vi "Discovery Management.vi"(11 "CIFPluginManager in":refnum<class "CIFPluginManager.lvclass">) -> (0 "error out":errorcluster)   [LabVIEW 2021, in "CIFPluginManager.lvclass"]
uses:
  CIFPluginManager.lvclass
  typedef/Discover Command.ctl
  CIFUtilities/CIFLogs/CIFLogs.lvlib
  gRPC/CIF_Manager_Client_Wrapper/CIFManagerClientWrapper.lvlib
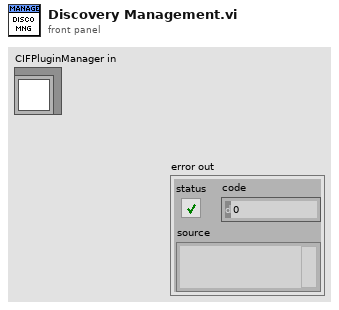
[diagram p1: front panel]
types:
  T1 = typedef "CIFPluginManager.lvclass/Discover Command.ctl" = cluster{"Loader Name":string, "Update Metadata":bool}
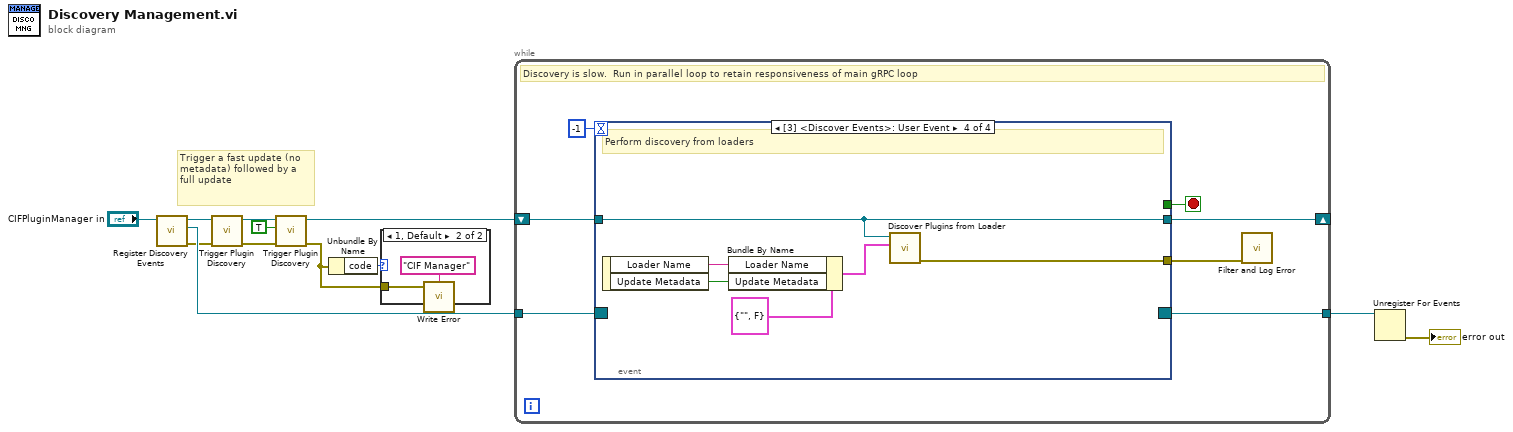
[diagram p0: block diagram]
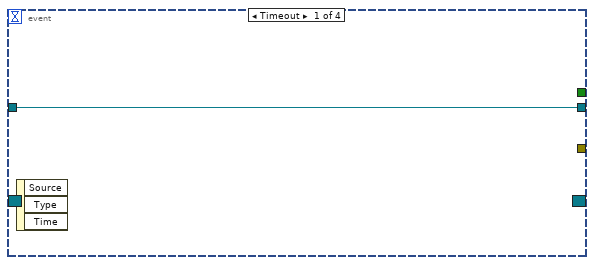
[diagram p3: hidden frame]
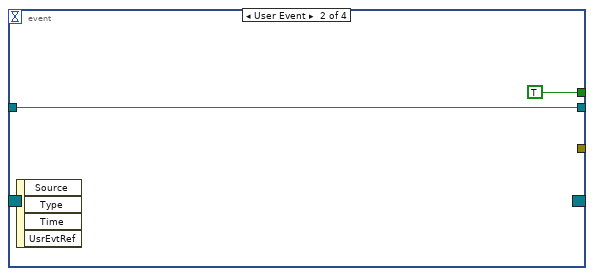
[diagram p4: hidden frame]
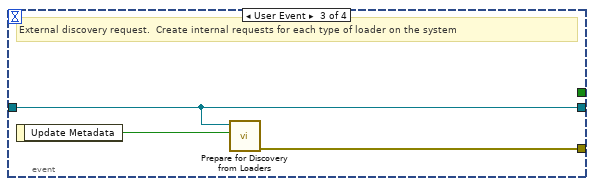
[diagram p5: hidden frame]
diagram:
  # "Trigger a fast update (no metadata) followed by a full update"
  n1 = call "Register Discovery Events.vi"("CIFPluginManager in"="CIFPluginManager in") -> ("error out"=w7:errorcluster, "Event Registration Refnum"=w9:refnum<event-registration>, "CIFPluginManager out"=w6:refnum<class "CIFPluginManager.lvclass">)  [unwired: 8 in]
  n2 = call "Trigger Plugin Discovery.vi"("error in (no error)"=w7, "CIFPluginManager in"=w6) -> ("error out"=w4:errorcluster, "CIFPluginManager out"=w5:refnum<class "CIFPluginManager.lvclass">)  [unwired: 8 in]
  n3 = call "Trigger Plugin Discovery.vi"("error in (no error)"=w4, "Update Metadata"=TRUE, "CIFPluginManager in"=w5) -> ("error out"=w2:errorcluster, "CIFPluginManager out"=w3:refnum<class "CIFPluginManager.lvclass">)  [unwired: 7 in]
  n4 = Unbundle By Name(w2) -> ("code"=w10:i32)
  n5 = case shown="1, Default" w10 {
    tunnel: w2 -> [_ w14]
    frame 0 {
      # "-1001 is cancelled by client.  Not an error."
    }
    frame 1, Default {
      n6 = call "Write Error.vi"("error in (no error)"=w14, "Plugin Name"="CIF Manager") -> ()  [unwired: 2 in, 1 out]
    }
  }
  n7 = while {
    tunnel: w9 -> [w15]
    shift-right: [w19] -> _
    shift-left: w3 -> [w21]
    tunnel: [w17] -> w11
    stop <- w18 stop-if-true
    # "Discovery is slow.  Run in parallel loop to retain responsiveness of main gRPC loop"
    n8 = event shown="[3] <Discover Events>: User Event" {
      selector: w15 -> [_ _ _ _]
      dyn-events: [_ _ _ _] -> w17
      timeout: -1 -> [_ _ _ _]
      tunnel: w21 -> [w22 w23 w26 w32]
      tunnel: [w22 w23 w26 w32] -> w19
      tunnel: [_ TRUE _ _] -> w18
      tunnel: [_ _ w25 w33] -> w16
      event Timeout {
        n9 = event-data() -> ()  [unwired: 1 in, 3 out]
      }
      event User Event {
        n10 = event-data() -> ()  [unwired: 1 in, 4 out]
      }
      event User Event {
        # "External discovery request.  Create internal requests for each type of loader on the system"
        n11 = event-data() -> ("Update Metadata"=w27:bool)  [unwired: 1 in]
        n12 = call "Prepare for Discovery from Loaders.vi"("Update Metadata"=w27, "CIFPluginManager in"=w26) -> ("error out"=w25:errorcluster)  [unwired: 9 in]
      }
      event User Event {
        # "Perform discovery from loaders"
        n13 = event-data() -> ("Loader Name"=w30:string, "Update Metadata"=w29:bool)  [unwired: 1 in]
        n14 = Bundle By Name(cluster=T1 {"Loader Name"="", "Update Metadata"=FALSE} ("Discovery Command"), "Loader Name"=w30, "Update Metadata"=w29) -> (w28:T1)
        n15 = call "Discover Plugins from Loader.vi"("Discovery Command"=w28, "CIFPluginManager in"=w32) -> ("error out"=w33:errorcluster)  [unwired: 9 in]
      }
    }
    n16 = call "Filter and Log Error.vi"("error In"=w16) -> ()  [unwired: 11 in]
  }
  n17 = Unregister For Events(event registration refnum=w11) -> (error out=→"error out":errorcluster)  [unwired: 1 in]
